vi "Set Default on UnInitialized INI Object.vi"(11 "ConfigManager.Text.INI":refnum<class "ConfigManager.Text.INI.lvclass">) -> (3 "ConfigManager.Text.INI":refnum<class "ConfigManager.Text.INI.lvclass">)   [LabVIEW 2013, in "CfgManager.Text.lvlib" / "ConfigManager.Text.INI.lvclass"]
uses:
  ConfigManager.Text.INI.lvclass
  Manager/ConfigManager.lvclass/ConfigManager.ctl
  <vilib>/LabVIEW Open Source Project/Serializer/Serializer/Serializer.lvclass
  <vilib>/LabVIEW Open Source Project/Unicity/Delimiter/Delimiter.lvclass
  <vilib>/LabVIEW Open Source Project/Serializer/Serializer.PlainText/Serializer.PlainText.lvclass
  Manager.Text/ConfigManager.Text.lvclass/ConfigManager.Text.ctl
  <vilib>/LabVIEW Open Source Project/Unicity/Delimiter/Delimiters List.ctl
  Manager/ConfigManager.lvclass
  Manager.Text/ConfigManager.Text.lvclass
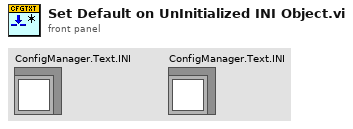
[diagram p1: front panel]
types:
  T1 = typedef "CfgManager.Text.lvlib/ConfigManager.Text.lvclass/Configuration -- Cluster.ctl" = cluster{"FileHeader":refnum<class "FileHeader.lvclass">, "FileSignature":refnum<class "FileSignature.lvclass">, "Section Delimiter":refnum<class "Delimiter.lvclass">, "Key-Value Separator":refnum<class "Delimiter.lvclass">}
  T2 = typedef "Delimiter.lvclass/Delimiters List.ctl" = enum16{"Default", "dot (.)", "colon (:)", "double-colon (::)", "semi-colon (;)", "underscore (_)", "double underscore (__)", "dash (-)", "double dash (--)", "backslash (\\)", "vertical bar (|)", "forward slash (/)", "chevron (>)", "double-chevron (>>)", "arrow (->)", "comma (,)", "arobas (@)", "ampersand (&)", "other"}
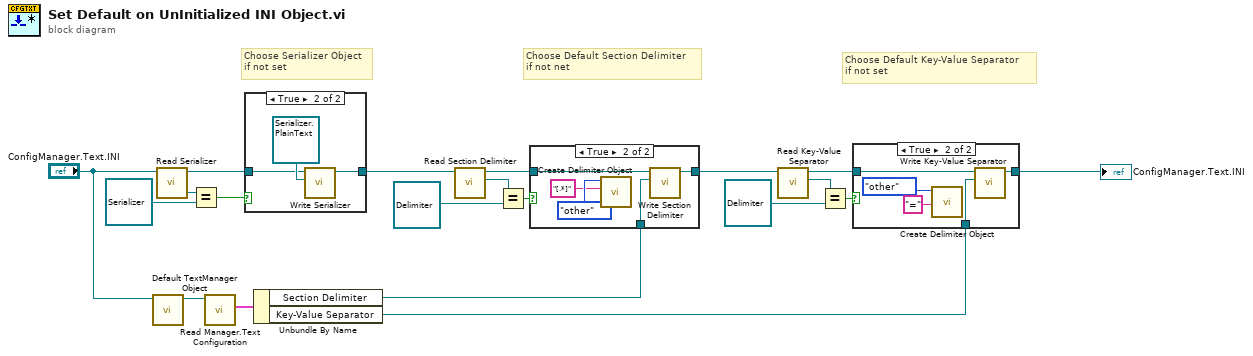
[diagram p0: block diagram]
diagram:
  # "Choose Default Key-Value Separator\nif not set"
  # "Choose Default Section Delimiter\nif not net"
  # "Choose Serializer Object\nif not set"
  n1 = call-dynamic "Default TextManager Object.vi"("CfgManager.Text in"="ConfigManager.Text.INI") -> ("CfgManager.Text out"=w5:refnum<class "ConfigManager.Text.INI.lvclass">)  [unwired: 10 in]
  n2 = call "Read Serializer.vi"("ConfigManager in"="ConfigManager.Text.INI") -> ("Serializer"=w12:refnum<class "Serializer.lvclass">, "ConfigManager out"=w11:refnum<class "ConfigManager.Text.INI.lvclass">)  [unwired: 9 in]
  n3 = Equal?(x=w12, y=refnum<class "Serializer.lvclass"> refnum) -> (x = y?=w14:bool)
  n4 = call "Read Manager.Text Configuration.vi"("ConfigManager.Text in"=w5) -> ("Manager.Text Configuration"=w4:T1)  [unwired: 9 in, 1 out]
  n5 = case shown="True" w14 {
    tunnel: [w21 w24] -> w19
    tunnel: w11 -> [w21 w22]
    frame False {
    }
    frame True {
      n6 = call "Write Serializer.vi"("Serializer"=refnum<class "Serializer.PlainText.lvclass"> refnum, "ConfigManager in"=w22) -> ("ConfigManager out"=w24:refnum<class "ConfigManager.Text.INI.lvclass">)  [unwired: 9 in]
    }
  }
  n7 = Unbundle By Name(w4) -> ("Section Delimiter"=w2:refnum<class "Delimiter.lvclass">, "Key-Value Separator"=w1:refnum<class "Delimiter.lvclass">)
  n8 = call "Read Section Delimiter.vi"("ConfigManager.Text in"=w19) -> ("Section Delimiter"=w17:refnum<class "Delimiter.lvclass">, "ConfigManager.Text out"=w15:refnum<class "ConfigManager.Text.INI.lvclass">)  [unwired: 9 in]
  n9 = Equal?(x=w17, y=refnum<class "Delimiter.lvclass"> refnum ("Key-Value Separator")) -> (x = y?=w20:bool)
  n10 = case shown="True" w20 {
    tunnel: w15 -> [w25 w30]
    tunnel: [w25 w29] -> w10
    tunnel: w2 -> [_ w27]
    frame False {
    }
    frame True {
      n11 = call <vilib>:"Create Delimiter Object.vi"("Other"="[.*]", "Delimiter"=Delimiters_List."other") -> ()  [unwired: 9 in, 1 out]
      n12 = call "Write Section Delimiter.vi"("Section Delimiter"=w27, "ConfigManager.Text in"=w30) -> ("ConfigManager.Text out"=w29:refnum<class "ConfigManager.Text.INI.lvclass">)  [unwired: 9 in]
    }
  }
  n13 = call "Read Key-Value Separator.vi"("ConfigManager.Text in"=w10) -> ("Key Value Separator"=w8:refnum<class "Delimiter.lvclass">, "ConfigManager.Text out"=w16:refnum<class "ConfigManager.Text.INI.lvclass">)  [unwired: 9 in]
  n14 = Equal?(x=w8, y=refnum<class "Delimiter.lvclass"> refnum ("Key-Value Separator")) -> (x = y?=w6:bool)
  n15 = case shown="True" w6 {
    tunnel: w16 -> [w31 w36]
    tunnel: [w31 w33] -> w9
    tunnel: w1 -> [_ w32]
    frame False {
    }
    frame True {
      n16 = call <vilib>:"Create Delimiter Object.vi"("Other"="=", "Delimiter"=Delimiters_List."other") -> ()  [unwired: 9 in, 1 out]
      n17 = call "Write Key-Value Separator.vi"("Key Value Delimiter"=w32, "ConfigManager.Text in"=w36) -> ("ConfigManager.Text out"=w33:refnum<class "ConfigManager.Text.INI.lvclass">)  [unwired: 9 in]
    }
  }
  "ConfigManager.Text.INI" <- w9
